vi "unmarshalling.vi"(7 "Type":variant, 8 "error in (no error)":errorcluster, 10 "XML String":string, 11 "Serializer":refnum<class "Serializer.easyXML.lvclass">) -> (0 "error out":errorcluster, 2 "Variant":variant, 3 "Serializer out":refnum<class "Serializer.easyXML.lvclass">)   [LabVIEW 2013, in "OpenSerializer.easyXML.lvlib" / "Serializer.easyXML.lvclass"]
uses:
  Serializer.easyXML.lvclass
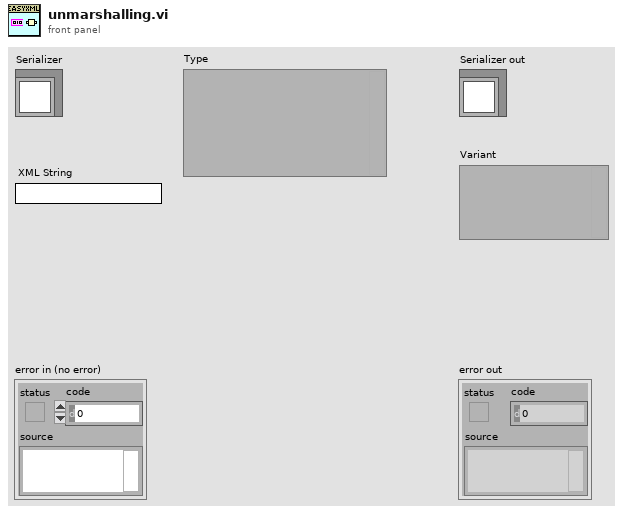
[diagram p1: front panel]
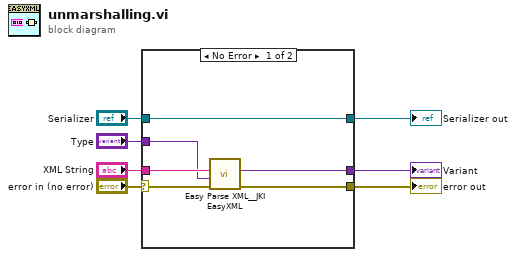
[diagram p0: block diagram]
diagram:
  n1 = case shown="No Error" "error in (no error)" {
    selector: "error in (no error)" -> [w10 w15]
    tunnel: "Serializer" -> [w13 w16]
    tunnel: "XML String" -> [w12 _]
    tunnel: [w13 w16] -> w5
    tunnel: [w9 w15] -> w4
    tunnel: [w11 w14] -> w3
    tunnel: "Type" -> [w8 w14]
    frame No Error {
      n2 = call <vilib>:"Easy Parse XML__JKI EasyXML.vi"("error in (no error)"=w10, "LabVIEW Data (Type)"=w8, "XML String"=w12) -> ("error out"=w9:errorcluster, "LabVIEW Data"=w11:variant)  [unwired: 7 in]
    }
    frame Error {
    }
  }
  "error out" <- w4
  "Serializer out" <- w5
  "Variant" <- w3
